vi "Draw Ends.vi"(0 "FSM.Edge In":refnum<class "FSM.Edge.lvclass">, 7 "picture in":picture) -> (4 "FSM.Edge Out":refnum<class "FSM.Edge.lvclass">, 8 "picture out":picture)   [LabVIEW 2020, in "FSM.Edge.lvclass"]
uses:
  FSM.Edge.lvclass
  FSM.Edge.lvclass/FSM.Edge.ctl
  FSM.EdgeEnd/FSM.EdgeEnd.lvclass
panel:
  out "error out":errorcluster
  in  "error in (no error)":errorcluster
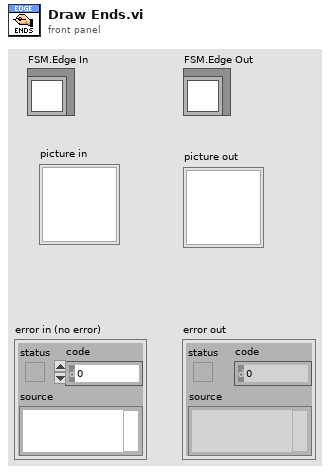
[diagram p1: front panel]
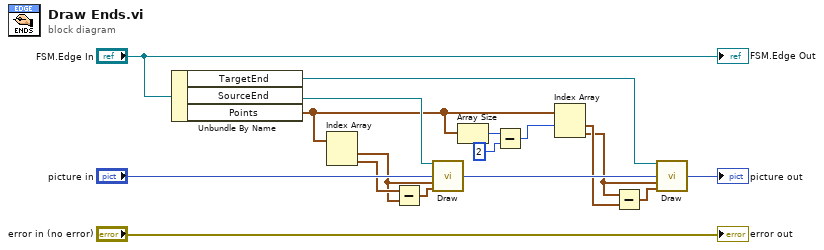
[diagram p0: block diagram]
diagram:
  n1 = Unbundle By Name("FSM.Edge In") -> ("TargetEnd"=w13:refnum<class "FSM.EdgeEnd.lvclass">, "SourceEnd"=w15:refnum<class "FSM.EdgeEnd.lvclass">, "Points"=w7:cluster{"x":i16, "y":i16}[])
  n2 = Index Array(array=w7) -> (element #1=w9:cluster{"x":i16, "y":i16}, element #2=w10:cluster{"x":i16, "y":i16})  [unwired: 2 in]
  n3 = Subtract(x=w10, y=w9) -> (x-y=w8:cluster{"x":i16, "y":i16})
  n4 = call "Draw.vi"("FSM.EdgeEnd"=w15, "picture in"="picture in", "location"=w9, "direction"=w8) -> ("picture out"=w12:picture)  [unwired: 11 in]
  n5 = Array Size(array=w7) -> (size(s)=w6:i32)
  n6 = Subtract(x=w6, y=2) -> (x-y=w4:i32)
  n7 = Index Array(array=w7, index #1=w4) -> (element #1=w3:cluster{"x":i16, "y":i16}, element #2=w2:cluster{"x":i16, "y":i16})  [unwired: 1 in]
  n8 = Subtract(x=w2, y=w3) -> (x-y=w1:cluster{"x":i16, "y":i16})
  n9 = call "Draw.vi"("FSM.EdgeEnd"=w13, "picture in"=w12, "location"=w2, "direction"=w1) -> ("picture out"=→"picture out":picture)  [unwired: 11 in]
  "FSM.Edge Out" <- "FSM.Edge In"
  "error out" <- "error in (no error)"
